vi "LineScan Preview the image.vi"() -> ()   [LabVIEW 2018]
uses:
  LabViewDVPCamera/LabViewDVPCamera.lvlib
  <vilib>/picture/picture.llb/imagedata.ctl
panel:
  in  "LineRate":u32=10 min=10 max=80000
  in  "LineTrigFreqDiv":u8
  in  "LineTrigFreqMult":u8
  in  "LineTrigFreqPreDiv":u8
  in  "LineTrigSource":enum16{"EncoderA", "EncoderB", "EncoderA&B"}(ring)
  out "Capture frame rate":sgl
  out "Total frame rate":u32
  out "pFrameCount out":T1
  out "frame rate":dbl format="%#.5g"
  out "number":u64
  out "Millisecond timing value 3":u32
  in  "image data":T2 caption="图像数据"
  in  "CloseFlg":i32
  out "handle":u32
  out "new picture":picture caption="新图片"
  in  "CameraList":u16(ring) items=["GLP4K4IR-H-192.168.10.37", "GLP4K4M-H-192.168.10.25", "GLP4K4M-H-192.168.10.57", "MGS502M-HO3-192.168.10.41", "MGS508-H2-169.254.10.254", "MGS508M-H2-192.168.10.61", "MGS508M-H22-192.168.10.54"]
  in  "Set":bool
  in  "Close":bool
  in  "Open":bool
  in  "ScanCamera":bool
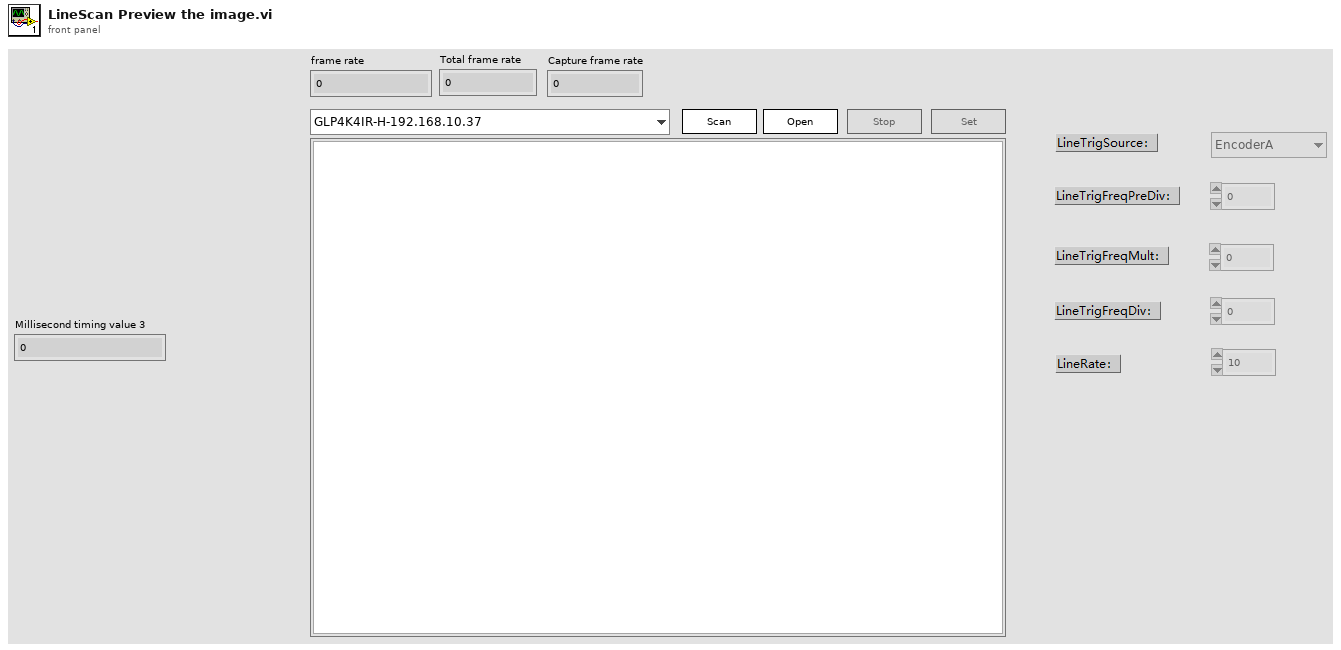
[diagram p1: front panel]
types:
  T1 = cluster{"uFrameCount":u32, "uFrameDrop":u32, "uFrameIgnore":u32, "uFrameError":u32, "uFrameOK":u32, "uFrameOut":u32, "uFrameResend":u32, "uFrameProc":u32, "fFrameRate":sgl, "fProcRate":sgl, "reserved[0]":i32, "reserved[1]":i32, "reserved[2]":i32, "reserved[3]":i32, "reserved[4]":i32, "reserved[5]":i32, "reserved[6]":i32, "reserved[7]":i32, "reserved[8]":i32, "reserved[9]":i32, "reserved[10]":i32, "reserved[11]":i32, "reserved[12]":i32, "reserved[13]":i32, "reserved[14]":i32, "reserved[15]":i32, "reserved[16]":i32, "reserved[17]":i32, "reserved[18]":i32, "reserved[19]":i32, "reserved[20]":i32, "reserved[21]":i32, "reserved[22]":i32, "reserved[23]":i32, "reserved[24]":i32, "reserved[25]":i32, "reserved[26]":i32, "reserved[27]":i32, "reserved[28]":i32, "reserved[29]":i32, "reserved[30]":i32, "reserved[31]":i32}
  T2 = typedef "imagedata.ctl" = cluster{"image type":i32, "image depth":i32, "image":u8[], "mask":u8[], "colors":u32[], "Rectangle":cluster{"left":i16, "top":i16, "right":i16, "bottom":i16}}
  T3 = enum8{"Enabled", "Disabled", "Disabled and Grayed Out"}
  T4 = typedef "LVStringsAndValuesArrayTypeDef_U16.ctl" = cluster{"String":string, "Value":u16}[]
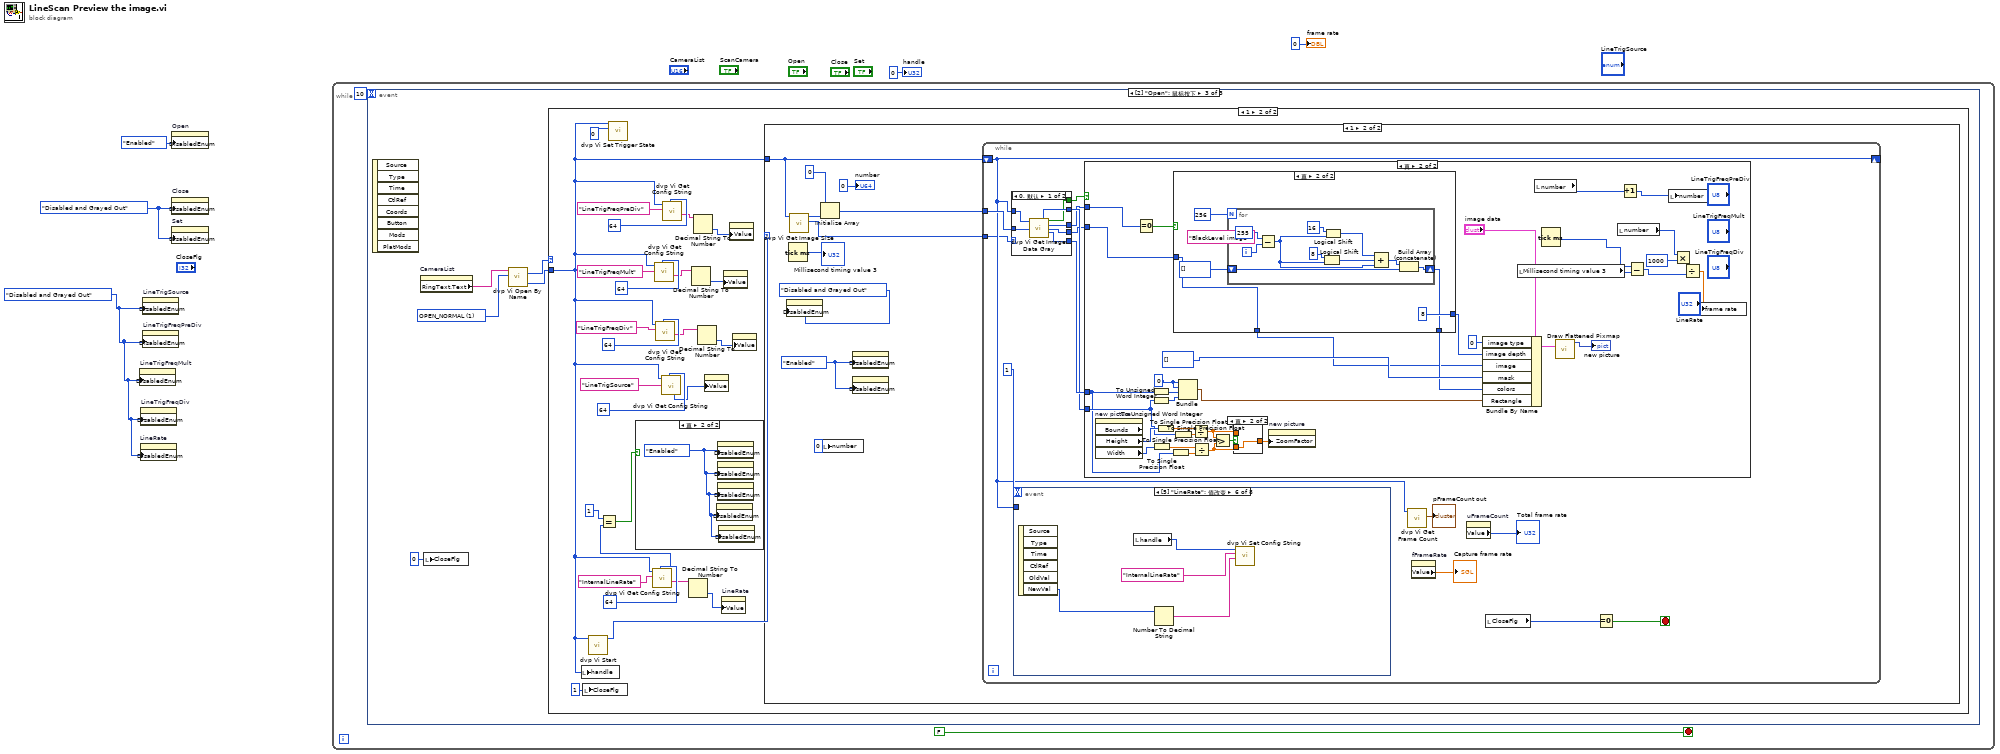
[diagram p0: block diagram]
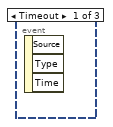
[diagram p2: hidden frame]
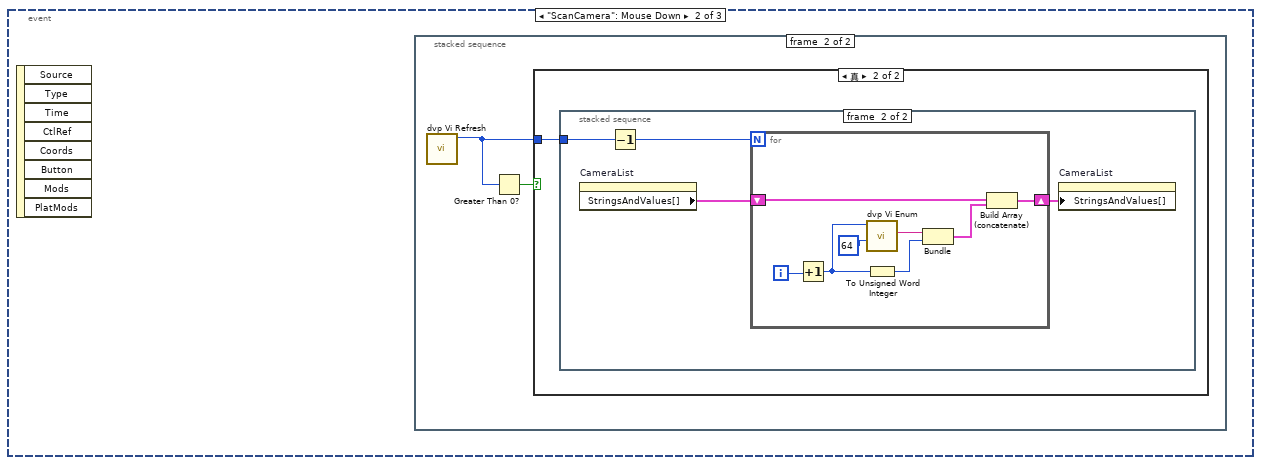
[diagram p3: hidden frame]
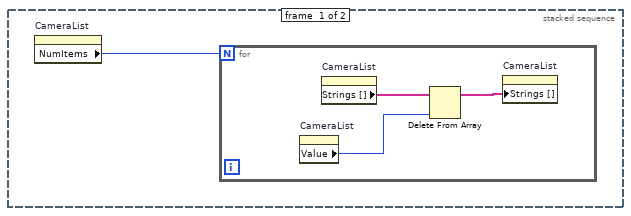
[diagram p4: hidden frame]
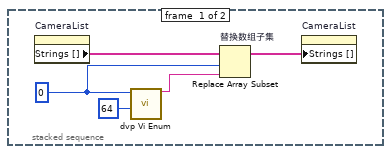
[diagram p6: hidden frame]
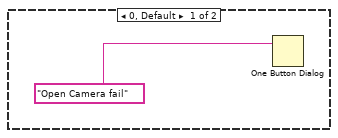
[diagram p7: hidden frame]
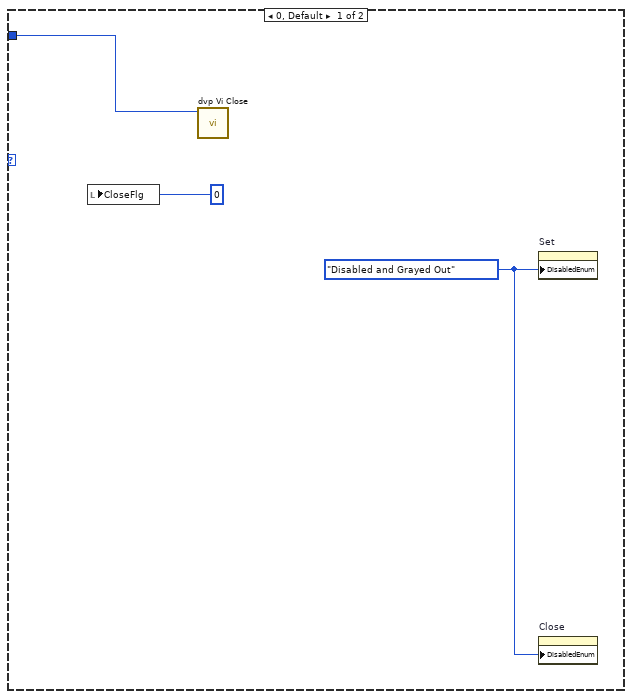
[diagram p9: hidden frame]
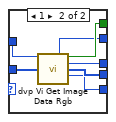
[diagram p10: hidden frame]
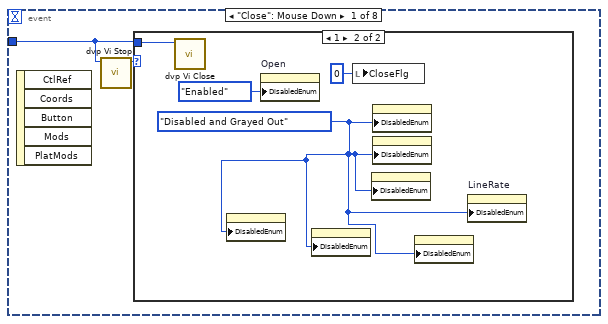
[diagram p11: hidden frame]
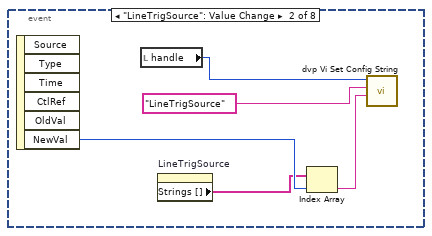
[diagram p13: hidden frame]
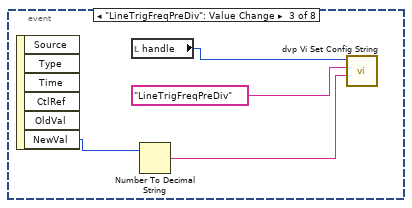
[diagram p14: hidden frame]
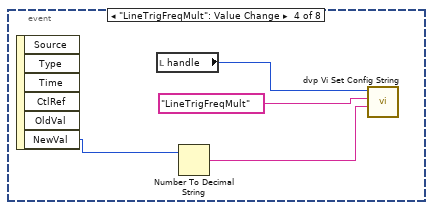
[diagram p15: hidden frame]
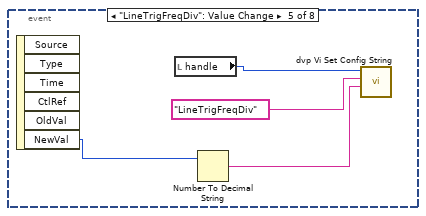
[diagram p16: hidden frame]
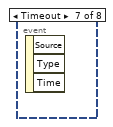
[diagram p17: hidden frame]
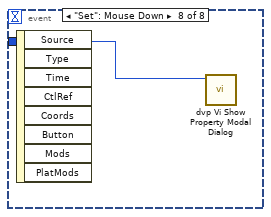
[diagram p18: hidden frame]
diagram:
  w1 = T3."Disabled and Grayed Out" ("禁用")
  w4 = T3."Disabled and Grayed Out" ("禁用")
  n1 = property on="LineTrigFreqMult" class="DigNum (严格)"("DisabledEnum"=w1) -> ()  [unwired: 2 in, 2 out]
  n2 = property on="LineRate" class="DigNum (严格)"("DisabledEnum"=w1) -> ()  [unwired: 2 in, 2 out]
  n3 = property on="LineTrigFreqDiv" class="DigNum (严格)"("DisabledEnum"=w1) -> ()  [unwired: 2 in, 2 out]
  n4 = property on="LineTrigSource" class="Enum (严格)"("DisabledEnum"=w1) -> ()  [unwired: 2 in, 2 out]
  n5 = property on="LineTrigFreqPreDiv" class="DigNum (严格)"("DisabledEnum"=w1) -> ()  [unwired: 2 in, 2 out]
  n6 = property on="Open" class="Bool"("DisabledEnum"=T3."Enabled" ("禁用")) -> ()  [unwired: 2 in, 2 out]
  n7 = property on="Close" class="Bool"("DisabledEnum"=w4) -> ()  [unwired: 2 in, 2 out]
  n8 = property on="Set" class="Bool"("DisabledEnum"=w4) -> ()  [unwired: 2 in, 2 out]
  n9 = while {
    stop <- FALSE stop-if-true
    n10 = event shown="[2] \"Open\": 鼠标按下" {
      selector: _ -> [_ _ _]
      dyn-events: _ -> [_ _ _]
      timeout: 10 -> [_ _ _]
      event Timeout {
        n11 = event-data() -> ()  [unwired: 1 in, 3 out]
      }
      event "ScanCamera": Mouse Down {
        n12 = event-data() -> ()  [unwired: 1 in, 8 out]
        n13 = stacked-sequence "清除下拉列表的数据" {
          frame #0 {
            n14 = property on="CameraList" class="Ring (严格)"() -> ("NumItems"=w8:u32)  [unwired: 2 in, 2 out]
            n15 = for {
              N: w8 -> [_]
              n16 = property on="CameraList" class="Ring (严格)"() -> ("Value"=w10:u16)  [unwired: 2 in, 2 out]
              n17 = property on="CameraList" class="Ring (严格)"() -> ("Strings []"=w9:string[])  [unwired: 2 in, 2 out]
              n18 = Delete From Array ("删除数组元素")(array=w9, index=w10) -> (array with subset deleted=w11:string[])  [unwired: 1 in, 1 out]
              n19 = property on="CameraList" class="Ring (严格)"("Strings []"=w11) -> ()  [unwired: 2 in, 2 out]
            }
          }
          frame #1 {
            n20 = call "dvp Vi Refresh.vi"() -> ("pCount out"=w13:u32)  [unwired: 10 in, 1 out]
            n21 = Greater Than 0?(x=w13) -> (x > 0?=w12:bool)
            n22 = case shown="真" w12 {
              tunnel: w13 -> [_ w14]
              frame False {
              }
              frame True {
                n23 = stacked-sequence {
                  tunnel: w14 -> [_ w21]
                  frame #0 {
                    w15 = u32 0 ("index")
                    n24 = property on="CameraList" class="Ring (严格)"() -> ("Strings []"=w18:string[])  [unwired: 2 in, 2 out]
                    n25 = call "dvp Vi Enum.vi"("unSize"=u32 64, "index"=w15) -> ("friendlyName out"=w17:string)  [unwired: 8 in, 1 out]
                    n26 = Replace Array Subset "替换数组子集"(array=w18, new element=w17, index=w15) -> (w19:string[])
                    n27 = property on="CameraList" class="Ring (严格)"("Strings []"=w19) -> ()  [unwired: 2 in, 2 out]
                  }
                  frame #1 {
                    n28 = property on="CameraList" class="Ring (严格)"() -> ("StringsAndValues[]"=w23:T4)  [unwired: 2 in, 2 out]
                    n29 = Decrement(x=w21) -> (x-1=w20:u32)
                    n30 = for {
                      N: w20 -> [_]
                      shift-right: [w30] -> w22
                      shift-left: w23 -> [w28]
                      i -> [w25]
                      n31 = Increment(x=w25) -> (x+1=w24:i32)
                      n32 = call "dvp Vi Enum.vi"("unSize"=u32 64, "index"=w24) -> ("friendlyName out"=w31:string)  [unwired: 8 in, 1 out]
                      n33 = To Unsigned Word Integer(number=w24) -> (unsigned 16bit integer=w27:u16)
                      n34 = Bundle("friendlyName out"=w31, w27) -> (w29:cluster{"friendlyName out":string, u16})  [unwired: 1 in]
                      n35 = Build Array (concatenate)(w28, w29) -> (w30:T4)
                    }
                    n36 = property on="CameraList" class="Ring (严格)"("StringsAndValues[]"=w22) -> ()  [unwired: 2 in, 2 out]
                  }
                }
              }
            }
          }
        }
      }
      event "Open": Mouse Down {
        w34 = u32 1 items=["OPEN_OFFLINE", "OPEN_NORMAL"] ("type")
        n37 = event-data() -> ()  [unwired: 1 in, 8 out]
        n38 = property on="CameraList" class="Ring (严格)"() -> ("RingText.Text"=w33:string)  [unwired: 2 in, 2 out]
        n39 = local write "CloseFlg"(0 ("CloseFlg")) -> ()
        n40 = call "dvp Vi Open By Name.vi"("type"=w34, "friendlyName"=w33) -> ("pHandle out"=w36:u32, "function return"=w35:u32)  [unwired: 7 in, 1 out]
        n41 = case shown="1" w35 {
          tunnel: w36 -> [_ w43]
          frame 0, Default {
            n42 = One Button Dialog(message="Open Camera fail" ("消息")) -> ()  [unwired: 1 in, 1 out]
          }
          frame 1 {
            n43 = local write "handle"(w43) -> ()
            n44 = local write "CloseFlg"(1 ("CloseFlg")) -> ()
            n45 = call "dvp Vi Start.vi"("handle"=w43) -> ("function return"=w62:u32)  [unwired: 10 in]
            n46 = call "dvp Vi Set Trigger State.vi"("TriggerState"=0, "handle"=w43) -> ()  [unwired: 9 in, 1 out]
            n47 = call "dvp Vi Get Config String.vi"("unSize"=64, "pszName"="InternalLineRate", "handle"=w43) -> ("pszValue out"=w58:string, "function return"=w55:u32)  [unwired: 5 in, 2 out]
            n48 = Equal?(x=1, y=w55) -> (x = y?=w54:bool)
            n49 = case shown="真" w54 {
              frame False {
              }
              frame True {
                w64 = T3."Enabled" ("禁用")
                n50 = property class="DigNum (严格)"("DisabledEnum"=w64) -> ()  [unwired: 2 in, 2 out]
                n51 = property class="DigNum (严格)"("DisabledEnum"=w64) -> ()  [unwired: 2 in, 2 out]
                n52 = property class="DigNum (严格)"("DisabledEnum"=w64) -> ()  [unwired: 2 in, 2 out]
                n53 = property class="DigNum (严格)"("DisabledEnum"=w64) -> ()  [unwired: 2 in, 2 out]
                n54 = property class="Enum (严格)"("DisabledEnum"=w64) -> ()  [unwired: 2 in, 2 out]
              }
            }
            n55 = call "dvp Vi Get Config String.vi"("unSize"=64, "pszName"="LineTrigFreqMult", "handle"=w43) -> ("pszValue out"=w45:string)  [unwired: 5 in, 3 out]
            n56 = call "dvp Vi Get Config String.vi"("unSize"=64, "pszName"="LineTrigFreqDiv", "handle"=w43) -> ("pszValue out"=w48:string)  [unwired: 5 in, 3 out]
            n57 = call "dvp Vi Get Config String.vi"("unSize"=64, "pszName"="LineTrigSource", "handle"=w43) -> ("pIndex out"=w51:u32)  [unwired: 5 in, 3 out]
            n58 = call "dvp Vi Get Config String.vi"("unSize"=64, "pszName"="LineTrigFreqPreDiv", "handle"=w43) -> ("pszValue out"=w40:string)  [unwired: 5 in, 3 out]
            n59 = Decimal String To Number(string=w58) -> (number=w57:i32)  [unwired: 2 in, 1 out]
            n60 = Decimal String To Number(string=w45) -> (number=w44:i32)  [unwired: 2 in, 1 out]
            n61 = Decimal String To Number(string=w40) -> (number=w39:i32)  [unwired: 2 in, 1 out]
            n62 = Decimal String To Number(string=w48) -> (number=w38:i32)  [unwired: 2 in, 1 out]
            n63 = property class="Enum (严格)"("Value"=w51) -> ()  [unwired: 2 in, 2 out]
            n64 = property on="LineRate" class="DigNum (严格)"("Value"=w57) -> ()  [unwired: 2 in, 2 out]
            n65 = property class="DigNum (严格)"("Value"=w44) -> ()  [unwired: 2 in, 2 out]
            n66 = property class="DigNum (严格)"("Value"=w39) -> ()  [unwired: 2 in, 2 out]
            n67 = property class="DigNum (严格)"("Value"=w38) -> ()  [unwired: 2 in, 2 out]
            n68 = case shown="1" w62 {
              tunnel: w43 -> [w67 w73]
              frame 0, Default {
                w66 = T3."Disabled and Grayed Out" ("禁用")
                n69 = local write "CloseFlg"(0 ("CloseFlg")) -> ()
                n70 = call "dvp Vi Close.vi"("handle"=w67) -> ()  [unwired: 10 in, 1 out]
                n71 = property on="Set" class="Bool"("DisabledEnum"=w66) -> ()  [unwired: 2 in, 2 out]
                n72 = property on="Close" class="Bool"("DisabledEnum"=w66) -> ()  [unwired: 2 in, 2 out]
              }
              frame 1 {
                w77 = T3."Enabled" ("禁用")
                n73 = property on="Open" class="Bool"("DisabledEnum"=T3."Disabled and Grayed Out" ("禁用")) -> ()  [unwired: 2 in, 2 out]
                n74 = Tick Count (ms)() -> (millisecond timer value=→"Millisecond timing value 3":u32)
                n75 = call "dvp Vi Get Image Size.vi"("handle"=w73) -> ("pformat out"=w69:i32, "function return"=w72:u32)  [unwired: 9 in]
                n76 = Initialize Array(u32 0 ("元素"), w72) -> (w74:u32[])
                n77 = local write "number"(u64 0 ("数值")) -> ()
                n78 = property on="Set" class="Bool"("DisabledEnum"=w77) -> ()  [unwired: 2 in, 2 out]
                n79 = property on="Close" class="Bool"("DisabledEnum"=w77) -> ()  [unwired: 2 in, 2 out]
                n80 = while {
                  shift-right: [w84] -> _
                  shift-left: w73 -> [w84]
                  tunnel: w74 -> [w85]
                  tunnel: w69 -> [w83]
                  stop <- w90 stop-if-true
                  n81 = case shown="0, 默认" w83 {
                    tunnel: w85 -> [w98 w105]
                    tunnel: w84 -> [w97 w104]
                    tunnel: [w93 w103] -> w79
                    tunnel: [w95 w102] -> w78
                    tunnel: [w94 w101] -> w80
                    tunnel: [w96 w100] -> w81
                    tunnel: [w92 w99] -> w82
                    frame 0, Default {
                      n82 = call "dvp Vi Get Image Data Gray.vi"("handle"=w97, "pbuffer"=w98) -> ("piHeight out"=w96:i32, "function return"=w93:bool, "pformat out"=w94:i32, "pbuffer out"=w95:u8[], "piWidth out"=w92:i32)  [unwired: 9 in]
                    }
                    frame 1 {
                      n83 = call "dvp Vi Get Image Data Rgb.vi"("handle"=w104, "pbuffer"=w105) -> ("piHeight out"=w100:i32, "function return"=w103:bool, "pformat out"=w101:i32, "pbuffer out"=w102:u32[], "piWidth out"=w99:i32)  [unwired: 9 in]
                    }
                  }
                  n84 = event shown="[5] \"LineRate\": 值改变" {
                    selector: _ -> [_ _ _ _ _ _ _ _]
                    dyn-events: _ -> [_ _ _ _ _ _ _ _]
                    timeout: 1 -> [_ _ _ _ _ _ _ _]
                    tunnel: w84 -> [w106 _ _ _ _ _ _ w133]
                    event "Close": Mouse Down {
                      n85 = event-data() -> ()  [unwired: 1 in, 5 out]
                      n86 = call "dvp Vi Stop.vi"("handle"=w106) -> ("function return"=w107:u32)  [unwired: 10 in]
                      n87 = case shown="1" w107 {
                        tunnel: w106 -> [_ w109]
                        frame 0, Default {
                        }
                        frame 1 {
                          w108 = T3."Disabled and Grayed Out" ("禁用")
                          n88 = call "dvp Vi Close.vi"("handle"=w109) -> ()  [unwired: 10 in, 1 out]
                          n89 = property class="DigNum (严格)"("DisabledEnum"=w108) -> ()  [unwired: 2 in, 2 out]
                          n90 = property on="Open" class="Bool"("DisabledEnum"=T3."Enabled" ("禁用")) -> ()  [unwired: 2 in, 2 out]
                          n91 = property class="DigNum (严格)"("DisabledEnum"=w108) -> ()  [unwired: 2 in, 2 out]
                          n92 = local write "CloseFlg"(0 ("CloseFlg")) -> ()
                          n93 = property class="Enum (严格)"("DisabledEnum"=w108) -> ()  [unwired: 2 in, 2 out]
                          n94 = property on="Close" class="Bool"("DisabledEnum"=w108) -> ()  [unwired: 2 in, 2 out]
                          n95 = property on="Set" class="Bool"("DisabledEnum"=w108) -> ()  [unwired: 2 in, 2 out]
                          n96 = property class="DigNum (严格)"("DisabledEnum"=w108) -> ()  [unwired: 2 in, 2 out]
                          n97 = property on="LineRate" class="DigNum (严格)"("DisabledEnum"=w108) -> ()  [unwired: 2 in, 2 out]
                        }
                      }
                    }
                    event "LineTrigSource": Value Change {
                      n98 = event-data() -> ("NewVal"=w114:enum16{"EncoderA", "EncoderB", "EncoderA&B"})  [unwired: 1 in, 5 out]
                      n99 = local read "handle"() -> (w116:u32)
                      n100 = property on="LineTrigSource" class="Enum (严格)"() -> ("Strings []"=w113:string[])  [unwired: 2 in, 2 out]
                      n101 = Index Array(array=w113, index=w114) -> (element=w112:string)
                      n102 = call "dvp Vi Set Config String.vi"("pszValue"=w112, "pszName"="LineTrigSource", "handle"=w116) -> ()  [unwired: 6 in, 3 out]
                    }
                    event "LineTrigFreqPreDiv": Value Change {
                      n103 = event-data() -> ("NewVal"=w120:u8)  [unwired: 1 in, 5 out]
                      n104 = local read "handle"() -> (w119:u32)
                      n105 = Number To Decimal String(number=w120) -> (decimal integer string=w117:string)  [unwired: 1 in]
                      n106 = call "dvp Vi Set Config String.vi"("pszValue"=w117, "pszName"="LineTrigFreqPreDiv", "handle"=w119) -> ()  [unwired: 6 in, 3 out]
                    }
                    event "LineTrigFreqMult": Value Change {
                      n107 = event-data() -> ("NewVal"=w122:u8)  [unwired: 1 in, 5 out]
                      n108 = local read "handle"() -> (w124:u32)
                      n109 = Number To Decimal String(number=w122) -> (decimal integer string=w121:string)  [unwired: 1 in]
                      n110 = call "dvp Vi Set Config String.vi"("pszValue"=w121, "pszName"="LineTrigFreqMult", "handle"=w124) -> ()  [unwired: 6 in, 3 out]
                    }
                    event "LineTrigFreqDiv": Value Change {
                      n111 = event-data() -> ("NewVal"=w125:u8)  [unwired: 1 in, 5 out]
                      n112 = local read "handle"() -> (w128:u32)
                      n113 = Number To Decimal String(number=w125) -> (decimal integer string=w126:string)  [unwired: 1 in]
                      n114 = call "dvp Vi Set Config String.vi"("pszValue"=w126, "pszName"="LineTrigFreqDiv", "handle"=w128) -> ()  [unwired: 6 in, 3 out]
                    }
                    event "LineRate": Value Change {
                      n115 = event-data() -> ("NewVal"=w130:u32)  [unwired: 1 in, 5 out]
                      n116 = local read "handle"() -> (w132:u32)
                      n117 = Number To Decimal String(number=w130) -> (decimal integer string=w129:string)  [unwired: 1 in]
                      n118 = call "dvp Vi Set Config String.vi"("pszValue"=w129, "pszName"="InternalLineRate", "handle"=w132) -> ()  [unwired: 6 in, 3 out]
                    }
                    event Timeout {
                      n119 = event-data() -> ()  [unwired: 1 in, 3 out]
                    }
                    event "Set": Mouse Down {
                      n120 = event-data() -> ()  [unwired: 1 in, 8 out]
                      n121 = call "dvp Vi Show Property Modal Dialog.vi"("handle"=w133) -> ()  [unwired: 10 in, 1 out]
                    }
                  }
                  n122 = case shown="真" w79 {
                    tunnel: w78 -> [_ w136]
                    tunnel: w82 -> [_ w137]
                    tunnel: w81 -> [_ w138]
                    tunnel: w80 -> [_ w166]
                    frame False {
                    }
                    frame True {
                      w169 = u16 0
                      n123 = property on="new picture" class="Pict" props=["Bounds", "Height", "Width"]() -> ("Height"=w139:u32, "Width"=w140:u32)  [unwired: 2 in, 3 out]
                      n124 = Equal To 0?(x=w166) -> (x = 0?=w165:bool)
                      n125 = To Unsigned Word Integer(number=w137) -> (unsigned 16bit integer=w168:u16)
                      n126 = To Unsigned Word Integer(number=w138) -> (unsigned 16bit integer=w167:u16)
                      n127 = To Single Precision Float(number=w140) -> (single precision float=w147:sgl)
                      n128 = To Single Precision Float(number=w139) -> (single precision float=w141:sgl)
                      n129 = To Single Precision Float(number=w137) -> (single precision float=w143:sgl)
                      n130 = case shown="真" w165 {
                        tunnel: [32 u8 8 ("image depth")] -> w162
                        tunnel: [i32[] [] ("数组") w178] -> w160
                        tunnel: w136 -> [w173 w177]
                        tunnel: [w172 w177] -> w135
                        frame False {
                          n131 = Type Cast(type=u8[] [], x=w173) -> (*(type *) &x=w172:u8[])
                        }
                        frame True {
                          (unwired) "BlackLevel image"
                          n132 = for {
                            N: 256 -> [_]
                            shift-right: [w186] -> w178
                            shift-left: i32[] [] ("数组") -> [w185]
                            i -> [w182]
                            n133 = Subtract(x=255, y=w182) -> (x-y=w183:i32)
                            n134 = Logical Shift(y=i16 8, x=w183) -> (x << y=w188:i32)
                            n135 = Logical Shift(y=16 ("x"), x=w183) -> (x << y=w189:i32)
                            n136 = Compound Arithmetic op=ADD(w189, w188, w183) -> (w187:i32)
                            n137 = Build Array (concatenate)(w187, w185) -> (w186:i32[])
                          }
                        }
                      }
                      n138 = To Single Precision Float(number=w138) -> (single precision float=w142:sgl)
                      n139 = Bundle ("图像尺寸")(w169, w169, w168, w167) -> (w159:cluster{u16, u16, u16, u16})  [unwired: 1 in]
                      n140 = Divide(x=w141, y=w142) -> (x/y=w145:sgl)
                      n141 = Divide(x=w147, y=w143) -> (x/y=w146:sgl)
                      n142 = Greater?(x=w145, y=w146) -> (0:w144:bool)
                      n143 = case shown="真" w144 {
                        tunnel: w145 -> [w170 _]
                        tunnel: w146 -> [_ w171]
                        tunnel: [w170 w171] -> w148
                        frame False {
                        }
                        frame True {
                        }
                      }
                      n144 = property on="new picture" class="Pict"("ZoomFactor"=w148) -> ()  [unwired: 2 in, 2 out]
                      n145 = Bundle By Name(cluster="image data", "image type"=0, "image depth"=w162, "image"=w135, "mask"=u8[] [] ("无符号8位数组"), "colors"=w160, "Rectangle"=w159) -> (w163:T2)
                      n146 = local read "Millisecond timing value 3"() -> (w151:u32)
                      n147 = local read "number"() -> (w154:u64)
                      n148 = Tick Count (ms)() -> (millisecond timer value=w152:u32)
                      n149 = call <vilib>:"Draw Flattened Pixmap.vi"("image data"=w163) -> ("new picture"=→"new picture":picture)  [unwired: 8 in]
                      n150 = local read "number"() -> (w150:u64)
                      n151 = Increment(x=w154) -> (x+1=w153:u64)
                      n152 = Subtract(x=w152, y=w151) -> (x-y=w157:u32)
                      n153 = local write "number"(w153) -> ()
                      n154 = Multiply(x=w150, y=u64 1000) -> (x*y=w155:u64)
                      n155 = Divide(x=w155, y=w157) -> (x/y=w149:dbl)
                      n156 = local write "frame rate"(w149) -> ()
                    }
                  }
                  n157 = call "dvp Vi Get Frame Count.vi"("handle"=w84) -> ("pFrameCount out"=→"pFrameCount out":T1)  [unwired: 9 in, 1 out]
                  n158 = property on="fFrameRate" class="DigNum (严格)"() -> ("Value"=→"Capture frame rate":sgl)  [unwired: 2 in, 2 out]
                  n159 = property on="uFrameCount" class="DigNum (严格)"() -> ("Value"=→"Total frame rate":u32)  [unwired: 2 in, 2 out]
                  n160 = local read "CloseFlg"() -> (w89:i32)
                  n161 = Equal To 0?(x=w89) -> (x = 0?=w90:bool)
                }
                "number" <- u64 0
              }
            }
          }
        }
      }
    }
  }
  "handle" <- u32 0 ("handle")
  "frame rate" <- 0
